vi "CT_PWM_Append.vi"(9 "PWM Enable":bool[](array[boolean]), 10 "PWM Level":u16[](array[numeric]), 11 "Duration":u16) -> (2 "Appended PWM Level":u16[](array[numeric]), 3 "Appended Duration Array":u16[](array[numeric]))   [LabVIEW 2016]
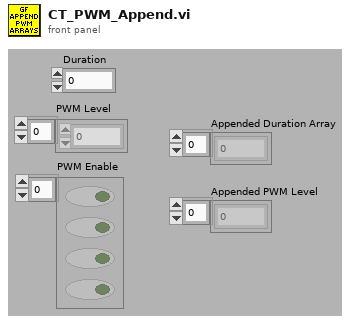
[diagram p1: front panel]
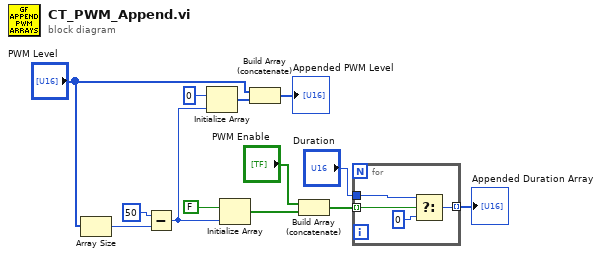
[diagram p0: block diagram]
diagram:
  n1 = Array Size(array="PWM Level") -> (size(s)=w13:i32)
  n2 = Subtract(x=50 ("dimension size"), y=w13) -> (x-y=w10:i32)
  n3 = Initialize Array(u16 0 ("dimension size"), w10) -> (w9:u16[])
  n4 = Initialize Array(FALSE, w10) -> (w8:bool[])
  n5 = Build Array (concatenate)("PWM Level", w9) -> (→"Appended PWM Level":u16[])
  n6 = Build Array (concatenate)("PWM Enable", w8) -> (w3:bool[])
  n7 = for {
    tunnel: w3 -> [w17] mode=indexing
    tunnel: "Duration" -> [w16]
    tunnel: [w14] -> w1 mode=indexing
    n8 = Select(t=w16, s=w17, f=u16 0) -> (s? t:f=w14:u16)
  }
  "Appended Duration Array" <- w1
